vi "DrawBarPlot.vi"(0 "reference in":refnum<class "HTMLPlot.lvclass">, 1 "XLabels":string[](array[string]), 2 "BarPlot.Dataset":dbl[][](array[numeric]), 3 "BarPlot.DatasetLabels":string[](array[string]), 5 "error in (no error)":errorcluster, 6 "GenericPlotOptions":T1, 7 "BarPlot.PlotColours":u32[](array[numeric]), 8 "BarPlotOptions":T3={"xLabel"="", "yLabel"="", "DisplayXLabel"=TRUE, "DisplayYLabel"=TRUE, "Stacked"=TRUE}) -> (14 "reference out":refnum<class "HTMLPlot.lvclass">, 19 "error out":errorcluster)   [LabVIEW 2019, in "HTMLPlot.lvclass"]
uses:
  HTMLPlot.lvclass
  Controls/GenericPlotOptions.ctl
  Controls/LegendPosition.ctl
  Controls/BarPlotOptions.ctl
panel:
  in  "LegendPosition":T2=enum."right"
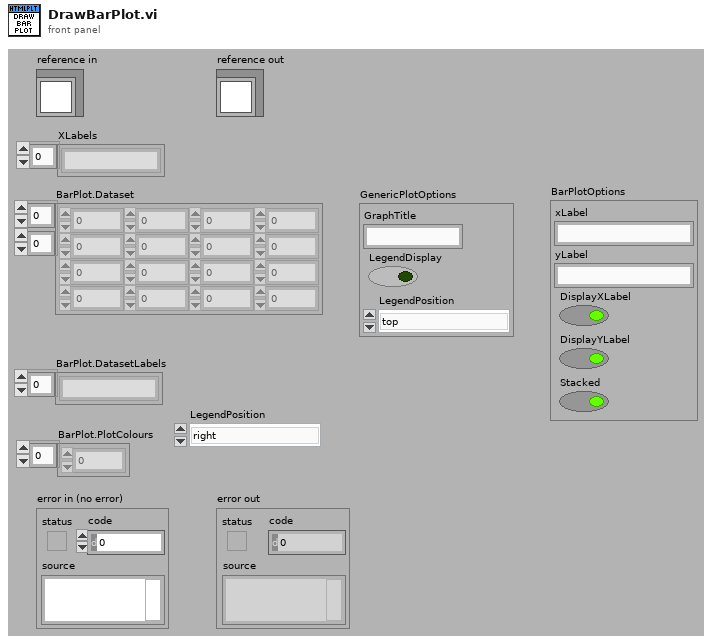
[diagram p1: front panel]
types:
  T1 = typedef "HTMLPlot.lvclass/GenericPlotOptions.ctl" = cluster{"GraphTitle":string, "LegendDisplay":bool, "LegendPosition":T2}
  T2 = typedef "HTMLPlot.lvclass/LegendPosition.ctl" = enum16{"top", "right", "left", "bottom"}
  T3 = typedef "HTMLPlot.lvclass/BarPlotOptions.ctl" = cluster{"xLabel":string, "yLabel":string, "DisplayXLabel":bool, "DisplayYLabel":bool, "Stacked":bool}
  T4 = cluster{"action":string, "PlotData":string, "GenericPlotOptions":T1, "BarPlotOptions":T3}
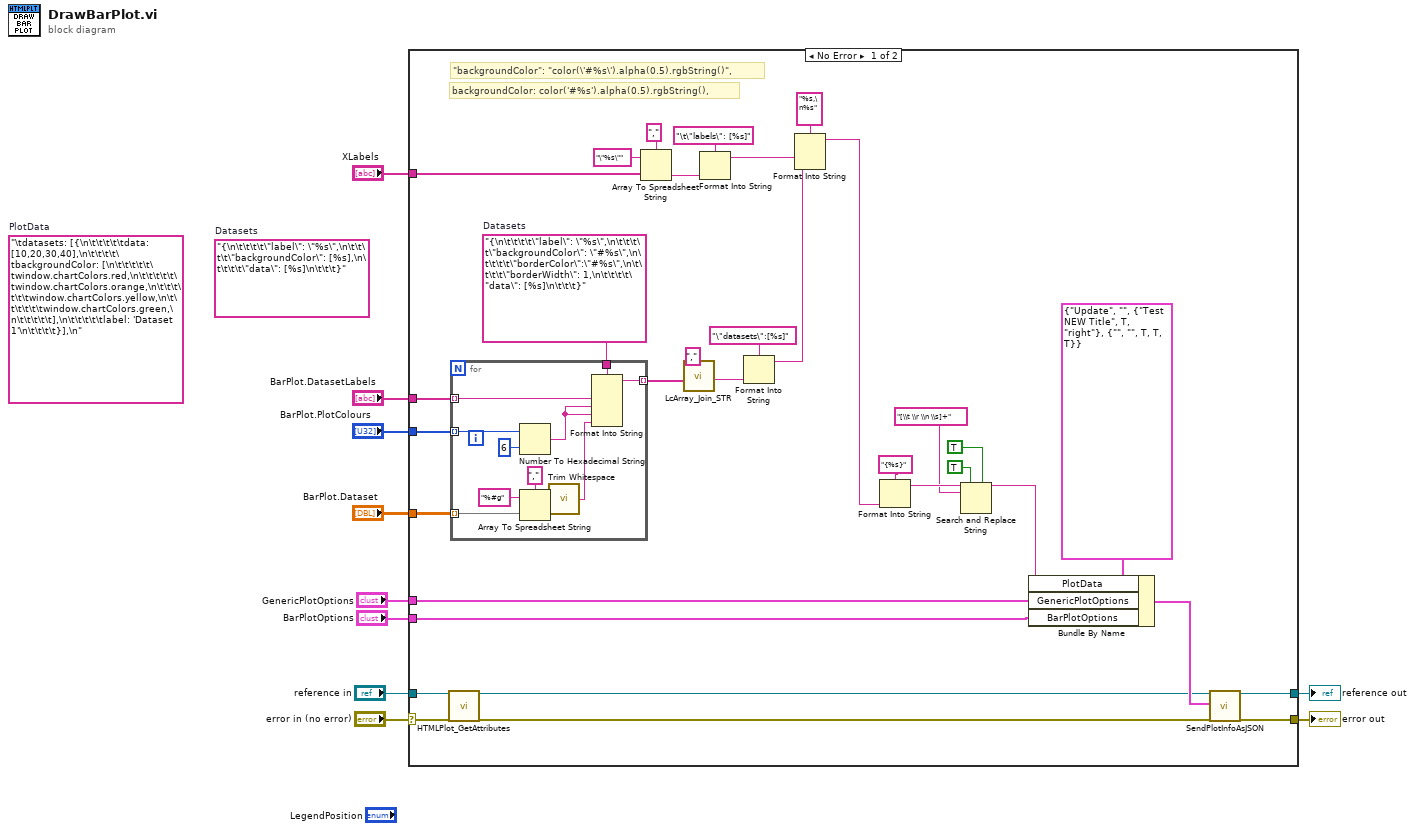
[diagram p0: block diagram]
diagram:
  (unwired) "{\n\t\t\t\t\"label\": \"%s\",\n\t\t\t\t\"backgroundColor\": [%s],\n\t\t\t\t\"data\": [%s]\n\t\t\t}"  # Datasets
  (unwired) "\tdatasets: [{\n\t\t\t\t\tdata: [10,20,30,40],\n\t\t\t\t\tbackgroundColor: [\n\t\t\t\t\t\twindow.chartColors.red,\n\t\t\t\t\t\twindow.chartColors.orange,\n\t\t\t\t\t\twindow.chartColors.yellow,\n\t\t\t\t\t\twindow.chartColors.green,\n\t\t\t\t\t],\n\t\t\t\t\tlabel: 'Dataset 1'\n\t\t\t\t}],\n"  # PlotData
  n1 = case shown="No Error" "error in (no error)" {
    selector: "error in (no error)" -> [w43 w56]
    tunnel: [w15 w56] -> w9
    tunnel: [w13 w55] -> w7
    tunnel: "reference in" -> [w42 w55]
    tunnel: "BarPlot.Dataset" -> [w29 _]
    tunnel: "BarPlot.PlotColours" -> [w28 _]
    tunnel: "BarPlot.DatasetLabels" -> [w27 _]
    tunnel: "XLabels" -> [w26 _]
    tunnel: "GenericPlotOptions" -> [w12 _]
    tunnel: "BarPlotOptions" -> [w11 _]
    frame No Error {
      w30 = "{\n\t\t\t\t\"label\": \"%s\",\n\t\t\t\t\"backgroundColor\": \"#%s\",\n\t\t\t\t\"borderColor\":\"#%s\",\n\t\t\t\t\"borderWidth\": 1,\n\t\t\t\t\"data\": [%s]\n\t\t\t}"  # Datasets
      # "\"backgroundColor\": \"color(\\'#%s\\').alpha(0.5).rgbString()\","
      # "backgroundColor: color('#%s').alpha(0.5).rgbString(),"
      n2 = call "HTMLPlot_GetAttributes.vi"("reference in"=w42, "error in (no error)"=w43) -> ("reference out"=w14:refnum<class "HTMLPlot.lvclass">, "error out"=w16:errorcluster)  [unwired: 14 in, 2 out]
      n3 = for {
        tunnel: w29 -> [w52] mode=indexing
        tunnel: w28 -> [w48] mode=indexing
        tunnel: w27 -> [w50] mode=indexing
        tunnel: [w49] -> w35 mode=indexing
        tunnel: w30 -> [w51]
        n4 = Number To Hexadecimal String(1:i16 6 ("width (-)"), 2:w48) -> (0:w47:string)
        n5 = Array To Spreadsheet String(delimiter (Tab)=",", array=w52, 3:"%#g" ("format string")) -> (spreadsheet string=w46:string)
        n6 = call <vilib>:"Trim Whitespace.vi"("string"=w46) -> ("trimmed string"=w45:string)  [unwired: 1 in]
        n7 = Format Into String(format string=w51, w50, w47, w47, w45) -> (resulting string=w49:string)  [unwired: 2 in, 1 out]
      }
      n8 = Array To Spreadsheet String(delimiter (Tab)=",", array=w26, 3:"\"%s\"" ("format string")) -> (spreadsheet string=w37:string)
      n9 = call "LcArray_Join_STR.vi"("separator"=",", "Array"=w35) -> ("joined string"=w34:string)  [unwired: 8 in, 1 out]
      n10 = Format Into String(format string="\t\"labels\": [%s]", w37) -> (resulting string=w40:string)  [unwired: 2 in, 1 out]
      n11 = Format Into String(format string="\"datasets\":[%s]", w34) -> (resulting string=w32:string)  [unwired: 2 in, 1 out]
      n12 = Format Into String(format string="%s,\n%s", w40, w32) -> (resulting string=w24:string)  [unwired: 2 in, 1 out]
      n13 = Format Into String(format string="{%s}", w24) -> (resulting string=w23:string)  [unwired: 2 in, 1 out]
      n14 = Search and Replace String(replace all?=TRUE ("replace all? (F)"), multiline?=TRUE ("multiline? (F)"), input string=w23, search string="[\\t \\r \\n \\s]+") -> (result string=w22:string)  [unwired: 4 in, 3 out]
      n15 = Bundle By Name(cluster=T4 {"action"="Update", "PlotData"="", "GenericPlotOptions"={"GraphTitle"="Test NEW Title", "LegendDisplay"=TRUE, "LegendPosition"=enum."right"}, "BarPlotOptions"={"xLabel"="", "yLabel"="", "DisplayXLabel"=TRUE, "DisplayYLabel"=TRUE, "Stacked"=TRUE}}, "PlotData"=w22, "GenericPlotOptions"=w12, "BarPlotOptions"=w11) -> (w17:T4)
      n16 = call "SendPlotInfoAsJSON.vi"("reference in"=w14, "PlotInfo"=w17, "error in (no error)"=w16) -> ("reference out"=w13:refnum<class "HTMLPlot.lvclass">, "error out"=w15:errorcluster)  [unwired: 15 in]
    }
    frame Error {
    }
  }
  "error out" <- w9
  "reference out" <- w7
